vi "APU Counters.vi"(7 "register bus":T1={"Speed"="Speed", "Crank Angle"="Crank Angle", "Cycle Angle"="Cycle Angle", "Crank Count"="Crank Count", "Cycle Count"="Cycle Count", "1.25 MHz Counter"="1.25 MHz Counter", "Crank Rollover"="Crank Rollover", "Cycle Rollover"="Cycle Rollover", "shared settings"={"start"=0.0, "stuck limit"=0.0}} {"shared settings"."start" format="%#.15g"}, 10 "reset":bool, 11 "actual speed":fxp<+/-,23,2>) -> (2 "cycle angle":u16, 3 "crank angle":u16)   [LabVIEW 2013, in "Engine Simulation Toolkit.lvlib" / "APU.lvlib"]
uses:
  APU.lvlib
  Register Bus.ctl
  Shared Settings.ctl
  Common/Count Up U5.vi
  <vilib>/rvi/DataTransferAndStorage/Container/Common/niFpgaContainerExecOnDevCompGetState.vi
  <vilib>/rvi/DataTransferAndStorage/Register/Emulation/niFpgaRegisterEmulationFpgaImpl.vi
  <instcachedir>/0/niFpgaRegisterEmulationFpgaImpl_DCF4BC0110594B98B44A971D60CEEC4D.lvgen/niFpgaRegisterEmulationFpgaImpl_DCF4BC0110594B98B44A971D60CEEC4D_018.vi
  <vilib>/rvi/DataTransferAndStorage/Container/Common/niFpgaContainerGetUniqueNameForEmu.vi
  <instcachedir>/0/niFpgaRegisterEmulationFpgaImpl_DCF4BC0110594B98B44A971D60CEEC4D.lvgen/niFpgaRegisterEmulationFpgaImpl_DCF4BC0110594B98B44A971D60CEEC4D_005.vi
  <instcachedir>/0/niFpgaRegisterEmulationFpgaImpl_DCF4BC0110594B98B44A971D60CEEC4D.lvgen/niFpgaRegisterEmulationFpgaImpl_DCF4BC0110594B98B44A971D60CEEC4D_006.vi
  <instcachedir>/0/niFpgaRegisterEmulationFpgaImpl_DCF4BC0110594B98B44A971D60CEEC4D.lvgen/niFpgaRegisterEmulationFpgaImpl_DCF4BC0110594B98B44A971D60CEEC4D_007.vi
  <instcachedir>/0/niFpgaRegisterEmulationFpgaImpl_DCF4BC0110594B98B44A971D60CEEC4D.lvgen/niFpgaRegisterEmulationFpgaImpl_DCF4BC0110594B98B44A971D60CEEC4D_008.vi
  <vilib>/rvi/DataTransferAndStorage/Container/XNode/niFpgaContainer.xnode
  <vilib>/rvi/DataTransferAndStorage/Register/Emulation/niFpgaRegisterEmulationRefIn.vi
  Engine Simulation Toolkit.lvlib
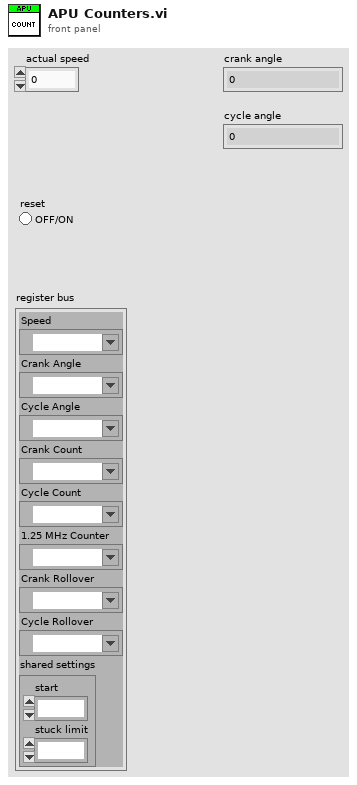
[diagram p1: front panel]
types:
  T1 = typedef "Engine Simulation Toolkit.lvlib/APU.lvlib/Register Bus.ctl" = cluster{"Speed":refnum<k21>, "Crank Angle":refnum<k21>, "Cycle Angle":refnum<k21>, "Crank Count":refnum<k21>, "Cycle Count":refnum<k21>, "1.25 MHz Counter":refnum<k21>, "Crank Rollover":refnum<k21>, "Cycle Rollover":refnum<k21>, "shared settings":T2}
  T2 = typedef "Engine Simulation Toolkit.lvlib/APU.lvlib/Shared Settings.ctl" = cluster{"start":fxp<+,17,17>, "stuck limit":fxp<+,18,18>}
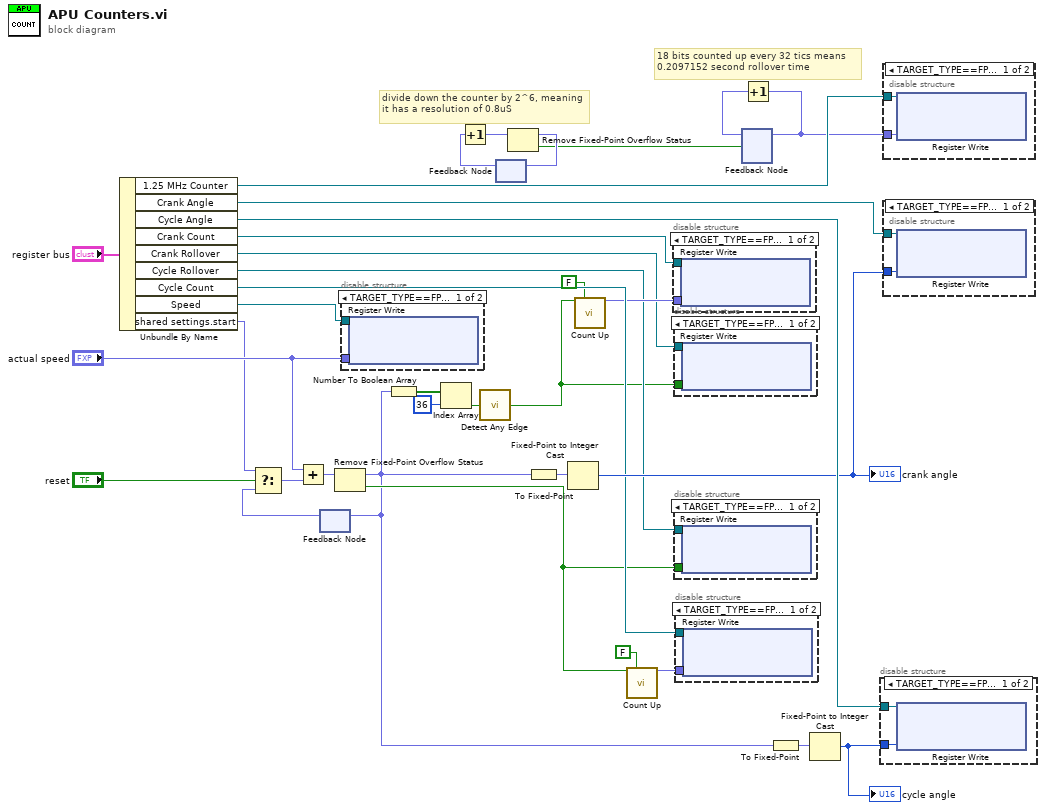
[diagram p0: block diagram]
diagram:
  # "18 bits counted up every 32 tics means\n0.2097152 second rollover time"
  # "divide down the counter by 2^6, meaning it has a resolution of 0.8uS"
  n1 = Unbundle By Name("register bus") -> ("1.25 MHz Counter"=w17:refnum<k21>, "Crank Angle"=w31:refnum<k21>, "Cycle Angle"=w32:refnum<k21>, "Crank Count"=w21:refnum<k21>, "Crank Rollover"=w8:refnum<k21>, "Cycle Rollover"=w7:refnum<k21>, "Cycle Count"=w24:refnum<k21>, "Speed"=w33:refnum<k21>, "shared settings.start"=w9:fxp<+,17,17>)
  n2 = feedback #1() -> (w35:fxp<+,37,17>)  [unwired: 1 in]
  n3 = Select(t=w9, s="reset", f=w35) -> (s? t:f=w30:fxp<+,37,17>)
  n4 = Add(x="actual speed", y=w30) -> (x+y=w28:fxp<+,37,17>)
  n5 = Remove Fixed-Point Overflow Status(3:w28) -> (0:w6:bool, 1:w1:fxp<+,37,17>)
  n6 = feedback-in #1(w1) -> ()
  n7 = disable-structure shown="TARGET_TYPE==FPGA" {
    disable-tunnel: w33 -> [w37 _]
    disable-tunnel: "actual speed" -> [w36 _]
    frame condition #0 (active) {
      n8 = xnode ("Register Write")("Data"=w36, "Register In"=w37) -> ()  [unwired: 1 out]
    }
    frame condition #1 {
    }
  }
  n9 = Number To Boolean Array(number=w1) -> (Boolean array=w5:bool[])
  n10 = Index Array(array=w5, index=36) -> (element=w3:bool)
  n11 = call "Detect Any Edge.vi"("signal"=w3) -> ("edge detected"=w2:bool)  [unwired: 14 in]
  n12 = feedback #2() -> (w15:fxp<+,5,5>)  [unwired: 1 in]
  n13 = Increment(x=w15) -> (x+1=w14:fxp<+,5,5>)
  n14 = Remove Fixed-Point Overflow Status(3:w14) -> (0:w12:bool, 1:w13:fxp<+,5,5>)
  n15 = feedback-in #2(w13) -> ()
  n16 = To Fixed-Point(number=w1) -> (fixed-point=w29:fxp<+,16,16>)  [unwired: 1 in]
  n17 = Fixed-Point to Integer Cast(1:w29) -> (0:w26:u16)
  "crank angle" <- w26
  n18 = call-poly "Count Up.vi"("increment"=w2, "reset"=FALSE) -> ("count out"=w22:fxp<+,5,5>)  [unwired: 13 in]
  n19 = call-poly "Count Up.vi"("increment"=w6, "reset"=FALSE) -> ("count out"=w20:fxp<+,5,5>)  [unwired: 13 in]
  n20 = disable-structure shown="TARGET_TYPE==FPGA" {
    disable-tunnel: w21 -> [w39 _]
    disable-tunnel: w22 -> [w38 _]
    frame condition #0 (active) {
      n21 = xnode ("Register Write")("Data"=w38, "Register In"=w39) -> ()  [unwired: 1 out]
    }
    frame condition #1 {
    }
  }
  n22 = disable-structure shown="TARGET_TYPE==FPGA" {
    disable-tunnel: w8 -> [w41 _]
    disable-tunnel: w2 -> [w40 _]
    frame condition #0 (active) {
      n23 = xnode ("Register Write")("Data"=w40, "Register In"=w41) -> ()  [unwired: 1 out]
    }
    frame condition #1 {
    }
  }
  n24 = disable-structure shown="TARGET_TYPE==FPGA" {
    disable-tunnel: w7 -> [w43 _]
    disable-tunnel: w6 -> [w42 _]
    frame condition #0 (active) {
      n25 = xnode ("Register Write")("Data"=w42, "Register In"=w43) -> ()  [unwired: 1 out]
    }
    frame condition #1 {
    }
  }
  n26 = disable-structure shown="TARGET_TYPE==FPGA" {
    disable-tunnel: w24 -> [w45 _]
    disable-tunnel: [w44 _] -> _
    disable-tunnel: w20 -> [w44 _]
    frame condition #0 (active) {
      n27 = xnode ("Register Write")("Data"=w44, "Register In"=w45) -> ()  [unwired: 1 out]
    }
    frame condition #1 {
    }
  }
  n28 = feedback #3() -> (w18:fxp<+,18,18>)  [unwired: 1 in]
  n29 = Increment(x=w18) -> (x+1=w16:fxp<+,18,18>)
  n30 = feedback-in #3(w16, w12) -> ()
  n31 = To Fixed-Point(number=w1) -> (fixed-point=w27:fxp<+,16,17>)  [unwired: 1 in]
  n32 = Fixed-Point to Integer Cast(1:w27) -> (0:w25:u16)
  "cycle angle" <- w25
  n33 = disable-structure shown="TARGET_TYPE==FPGA" {
    disable-tunnel: w32 -> [w47 _]
    disable-tunnel: w25 -> [w46 _]
    frame condition #0 (active) {
      n34 = xnode ("Register Write")("Data"=w46, "Register In"=w47) -> ()  [unwired: 1 out]
    }
    frame condition #1 {
    }
  }
  n35 = disable-structure shown="TARGET_TYPE==FPGA" {
    disable-tunnel: w17 -> [w49 _]
    disable-tunnel: w16 -> [w48 _]
    frame condition #0 (active) {
      n36 = xnode ("Register Write")("Data"=w48, "Register In"=w49) -> ()  [unwired: 1 out]
    }
    frame condition #1 {
    }
  }
  n37 = disable-structure shown="TARGET_TYPE==FPGA" {
    disable-tunnel: w31 -> [w51 _]
    disable-tunnel: w26 -> [w50 _]
    frame condition #0 (active) {
      n38 = xnode ("Register Write")("Data"=w50, "Register In"=w51) -> ()  [unwired: 1 out]
    }
    frame condition #1 {
    }
  }
